vi "DB Get Current Users.vi"(8 "error in (no error)":errorcluster) -> (0 "error out":errorcluster, 2 "Result (Rows or Columns)":string[](array[string]))   [LabVIEW 2019, in "Control Experiment.lvclass"]
uses:
  Control Experiment.lvclass
  <userlib>/LevyLab/LV-Data/LV-Data.PG/LV-Data.PGSQL.lvclass
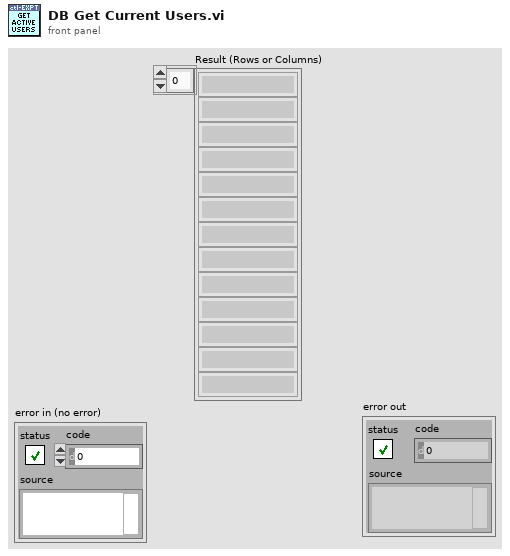
[diagram p1: front panel]
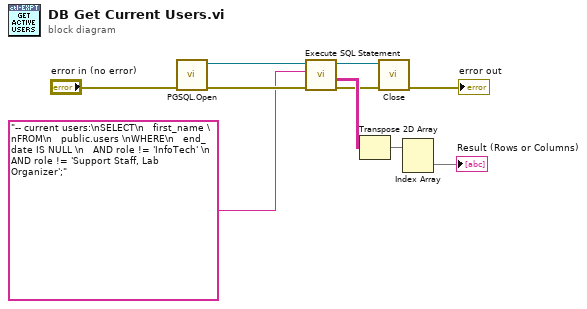
[diagram p0: block diagram]
diagram:
  n1 = call <userlib>:"PGSQL.Open.vi"("error in (no error)"="error in (no error)") -> ("error out"=w7:errorcluster, "Data.PG out"=w10:refnum<class "LV-Data.PGSQL.lvclass">)  [unwired: 9 in]
  n2 = call <userlib>:"Execute SQL Statement.vi"("error in (no error)"=w7, "SQL string"="-- current users:\nSELECT\n   first_name \nFROM\n   public.users \nWHERE\n   end_date IS NULL \n   AND role != 'InfoTech' \n   AND role != 'Support Staff, Lab Organizer';" ("Address"), "Data.PGQL in"=w10) -> ("error out"=w6:errorcluster, "Result"=w8:string[][], "Data.PGSQL out"=w9:refnum<class "LV-Data.PGSQL.lvclass">)  [unwired: 6 in]
  n3 = Transpose 2D Array(2D array=w8) -> (transposed array=w5:string[][])
  n4 = call-dynamic "Close.vi"("error in (no error)"=w6, "Data.PG in"=w9) -> ("error out"=→"error out":errorcluster)  [unwired: 8 in, 1 out]
  n5 = Index Array(array=w5) -> (element=→"Result (Rows or Columns)":string[])  [unwired: 2 in]
